vi "calcGaussianNextLineAddr.vi"(5 "preAddr":u16, 6 "divider":u8, 7 "Cols":u16, 9 "width":u16) -> (2 "nextAddr":u16)   [LabVIEW 2016]
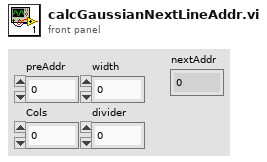
[diagram p1: front panel]
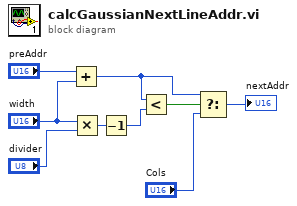
[diagram p0: block diagram]
diagram:
  n1 = Add(x="preAddr", y="width") -> (x+y=w4:u16)
  n2 = Multiply(x="width", y="divider") -> (x*y=w2:u16)
  n3 = Decrement(x=w2) -> (x-1=w1:u16)
  n4 = Less?(x=w4, y=w1) -> (x < y?=w8:bool)
  n5 = Select(t=w4, s=w8, f="Cols") -> (s? t:f=→"nextAddr":u16)
